vi "Convert R to T - DBL.vi"(8 "error in":errorcluster, 9 "R (kO)":dbl[](array[numeric])=[3.893, 10.0, 29.49], 10 "Tref (C)":dbl[](array[numeric])=[50.0, 25.0, 0.0], 11 "R":dbl caption="R (Ohms)") -> (0 "error out":errorcluster, 3 "T":dbl caption="T (degC)")   [LabVIEW 2015, in "Temperature.lvlib"]
doc: "Converts a thermistor resistance in kOhms to temperature a temperature in degrees Celsius."
uses:
  Temperature.lvlib
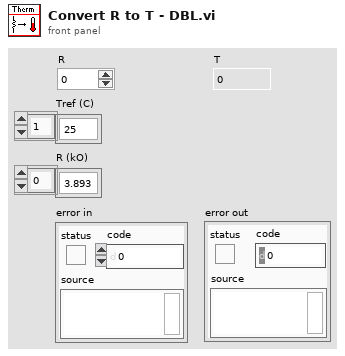
[diagram p1: front panel]
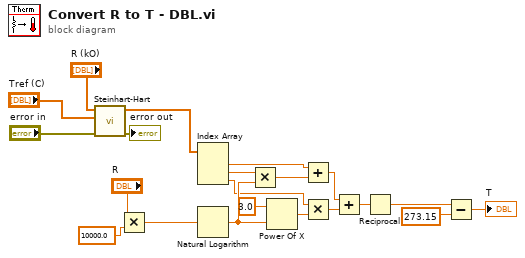
[diagram p0: block diagram]
diagram:
  n1 = call "Steinhart-Hart.vi"("error in"="error in", "Tref (C)"="Tref (C)", "R (kO)"="R (kO)") -> ("error out"=→"error out":errorcluster, "Coefficients"=w21:dbl[])  [unwired: 7 in]
  n2 = Multiply(x="R", y=10000.0) -> (x*y=w7:dbl)
  n3 = Index Array(array=w21) -> (element #1=w20:dbl, element #2=w18:dbl, element #3=w15:dbl)  [unwired: 3 in]
  n4 = Natural Logarithm(1:w7) -> (0:w17:dbl)
  n5 = Multiply(x=w18, y=w17) -> (x*y=w16:dbl)
  n6 = Power Of X(1:w17, 2:3.0 ("y")) -> (0:w14:dbl)
  n7 = Add(x=w20, y=w16) -> (x+y=w12:dbl)
  n8 = Multiply(x=w15, y=w14) -> (x*y=w13:dbl)
  n9 = Add(x=w12, y=w13) -> (x+y=w11:dbl)
  n10 = Reciprocal(x=w11) -> (1/x=w10:dbl)
  n11 = Subtract(x=w10, y=273.15) -> (x-y=→"T":dbl)
